vi "AFMss_control_trajTrack_deltaU_distEst.vi"() -> ()   [LabVIEW 2017]
uses:
  controls/controlParams_tracktraj.ctl
  <vilib>/rvi/Emulation/niFpgaGetClockAttributes.vi
  <vilib>/rvi/Emulation/niFpgaSctlEmulationGetInTimedLoop.vi
  <vilib>/rvi/Emulation/niFpgaEmulationReportErrorSimple.vi
  <vilib>/rvi/eio/common/nirviEmuTemplateMethod_errors.vi
  <vilib>/rvi/Emulation/niFpgaCriticalErrorInLSC.vi
  <vilib>/rvi/DataTransferAndStorage/Container/Common/niFpgaContainerExecOnDevCompGetState.vi
  <vilib>/rvi/Emulation/niFpgaEmulationIsFPGAContextNoSignature.vi
  <vilib>/rvi/DataTransferAndStorage/Container/Common/niFpgaContainerGetUniqueNameForEmu.vi
  <vilib>/rvi/Memory/Memory_Emulation/niFpgaMemoryEmulationCacheClearOnFirstRun.vi
  <vilib>/rvi/Memory/Memory_Emulation/nirvimemoryEmulationManagerCache_MakeExclusive.vi
  <vilib>/rvi/Memory/Memory_Emulation/niFpgaMemoryEmulationValidateCache.vi
  <vilib>/rvi/Memory/Memory_Emulation/nirvimemoryEmulationManagerCache_InsertValue.vi
  <vilib>/Utility/error.llb/Clear Errors.vi
  <vilib>/rvi/Memory/Memory_Emulation/nirvimemoryEmulationManagerCache_ReleaseExclusive.vi
  <vilib>/rvi/Memory/Memory_Emulation/nirvimemoryEmulationManagerCache_GetValue.vi
  <vilib>/rvi/Memory/Memory_Emulation/nirvimemoryEmulationManagerCache_SetValue.vi
  <vilib>/rvi/Emulation/niFpgaProcessEmulError.vi
  <vilib>/rvi/interface/RandomDataEmulation/niFpgaRandomDataHandleErrors.vi
  <vilib>/eio/EIONode/EIONode.xnode
  <vilib>/rvi/DataTransferAndStorage/Container/XNode/niFpgaContainer.xnode
  <vilib>/rvi/DataTransferAndStorage/Register/Emulation/niFpgaRegisterEmulationRefIn.vi
  <vilib>/rvi/interface/RandomDataEmulation/nirviRandomDataFpgaReadWriteTemplate.vi
  <vilib>/rvi/FXPMathLib/FxpSub/XNode/nifxpmath_Sub.xnode
  <vilib>/rvi/FXPMathLib/sim/FxpSim.dll
panel:
  in  "N_sat":i32
  in  "wsat_s":sgl[](array[numeric])=[0.0, 0.0, 0.0, 0.0, 0.0, 0.0, 0.0]
  in  "d_s":sgl[](array[numeric])=[0.0, 0.0, 0.0, 0.0, 0.0, 0.0, 0.0]
  in  "w_s":sgl[](array[numeric])=[0.0, 0.0, 0.0, 0.0, 0.0, 0.0, 0.0]
  in  "r_s":sgl[](array[numeric])=[0.0, 0.0, 0.0, 0.0, 0.0, 0.0, 0.0]
  in  "N_hyst":i32
  in  "Den":sgl[](array[numeric])=[0.982758, -1.98194, 1.0, 0.0, 0.0, 0.0, 0.0, 0.0, 0.0]
  in  "Num":sgl[](array[numeric])=[-0.00254, 0.000408, 0.00295, 0.0, 0.0, 0.0, 0.0, 0.0, 0.0]
  in  "TF Order":i32=2
  out "yk":sgl
  out "yuxk TO":bool
  out "YK TO":bool
  out "UK TO":bool
  in  "Cluster":T1={"umax"=3.0, "y_ref(k)"=0.0, "Ki"=0.0, "y(k) (from plant)"=0.0, "ND"=0, "NS"=0, "u_Kx_ref(k)"=0.0, "du_max"=3.0, "NS_obs"=0, "NS_control"=0, "Kp"=0.0} {"Kp" format="%#_13g"; "du_max" format="%#_13g"; "u_Kx_ref(k)" format="%#_13g"; "Ki" format="%#_13g"; "y_ref(k)" format="%#_13g"; "umax" format="%#_13g"}
  out "Unstable Traj":bool
  out "Loop Done":bool
  in  "Settle Ticks":i16=1000
  in  "False  = cont run":bool=TRUE
  in  "Abort":bool=TRUE
  in  "iters":i16=1
  in  "ymax":sgl=4.0 format="%#_13g"
  in  "TsTicks":i16
  out "Loop Ticks (benchmark)":i16
  out "NS_obs":i16=2
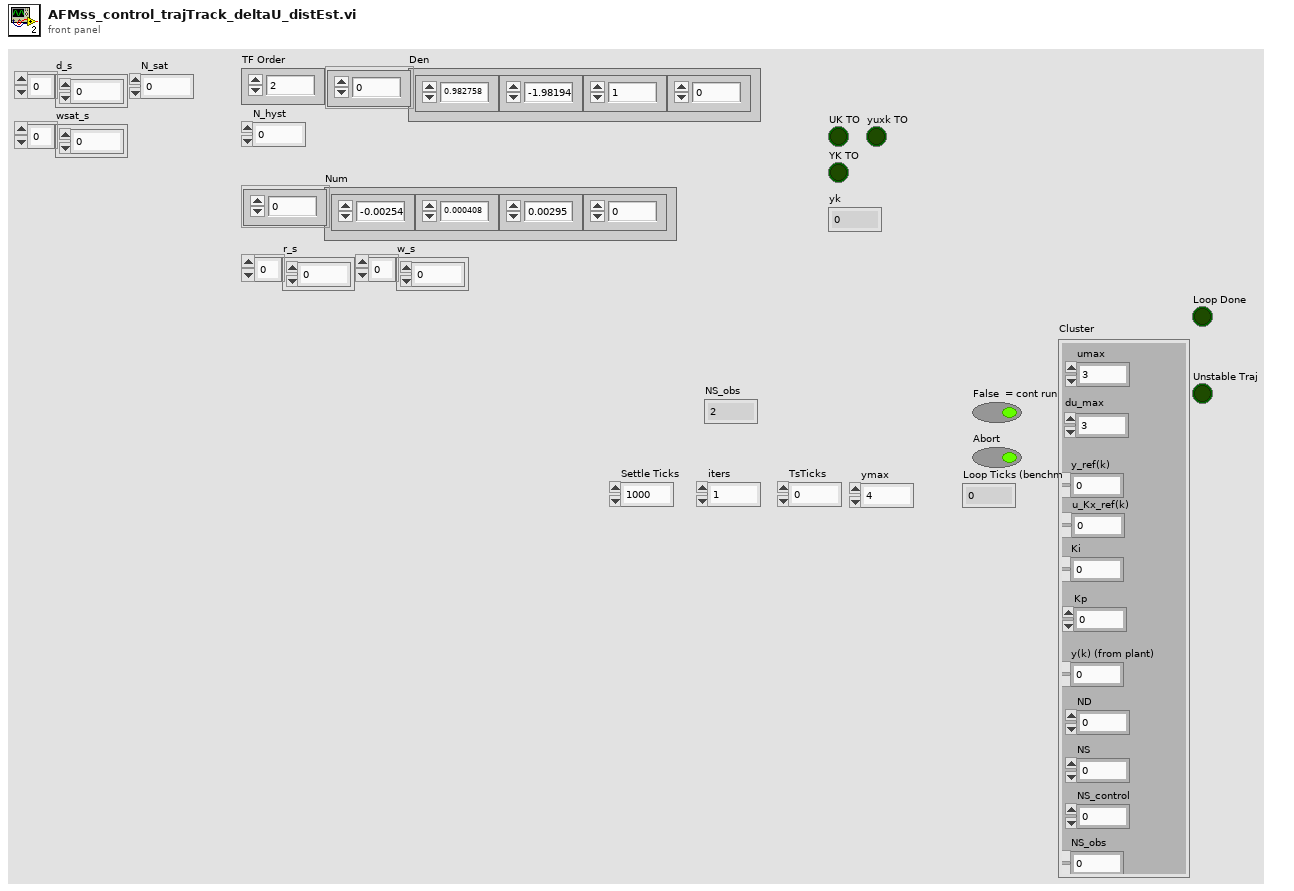
[diagram p1: front panel]
types:
  T1 = typedef "controlParams_tracktraj.ctl" = cluster{"umax":sgl, "y_ref(k)":sgl, "Ki":sgl, "y(k) (from plant)":sgl, "ND":i16, "NS":i16, "u_Kx_ref(k)":sgl, "du_max":sgl, "NS_obs":i16, "NS_control":i16, "Kp":sgl}
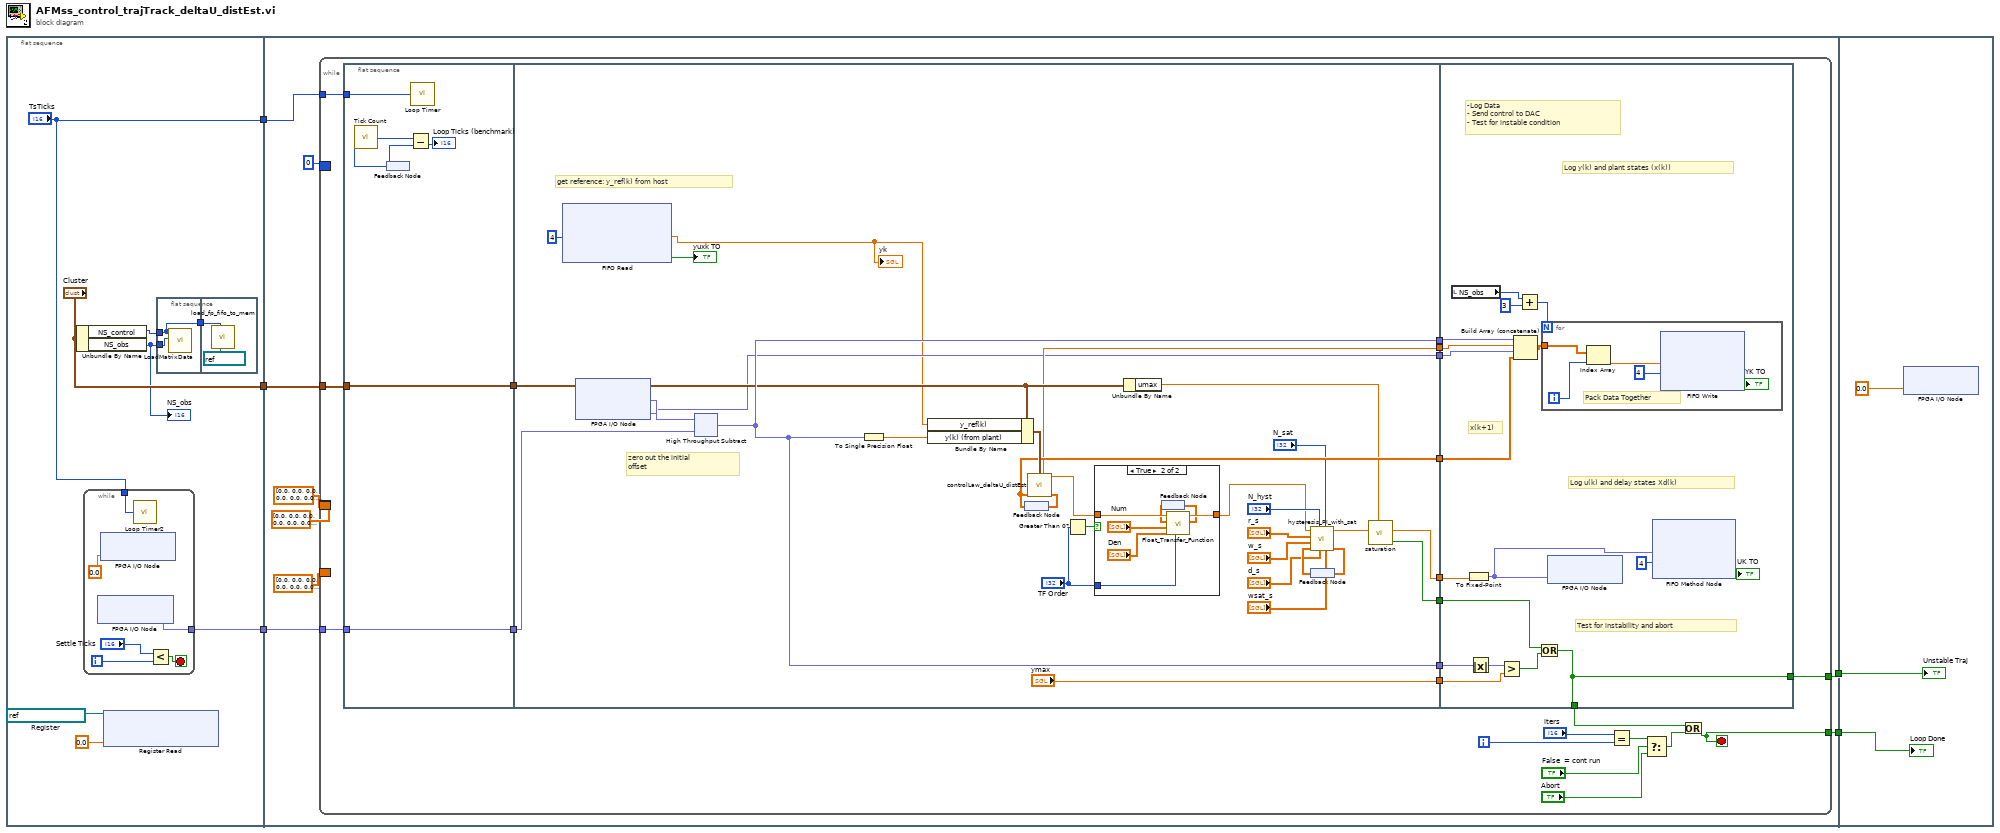
[diagram p0: block diagram]
diagram:
  n1 = flat-sequence {
    tunnel: ["TsTicks"] -> w5
    tunnel: [w13] -> w4
    tunnel: ["Cluster"] -> w2
    tunnel: w5 -> [w31]
    tunnel: w4 -> [w30]
    tunnel: [w29] -> w3
    tunnel: w2 -> [w28]
    tunnel: [w27] -> w1
    tunnel: w3 -> [w123]
    tunnel: w1 -> [w122]
    frame #0 {
      w11 = refnum<k21> "accumulator"  # Register
      # "Load Matrix Data"
      n2 = Unbundle By Name("Cluster") -> ("NS_control"=w8:i16, "NS_obs"=w6:i16)
      "NS_obs" <- w6
      n3 = while {
        tunnel: [w23] -> w13
        tunnel: "TsTicks" -> [w22]
        i -> [w18]
        stop <- w20 stop-if-true
        n4 = xnode "FPGA I/O Node"() -> ("Mod2/AI0"=w23:fxp<+/-,24,5>)  [unwired: 1 in, 1 out]
        n5 = xnode "FPGA I/O Node"("Mod1/AO0"=sgl 0.0) -> ()  [unwired: 1 in, 1 out]
        n6 = call "Loop Timer2"("Count(Ticks)"=w22) -> ()  [unwired: 1 out]
        n7 = Less?(x="Settle Ticks", y=w18) -> (x < y?=w20:bool)
      }
      n8 = xnode ("Register Read")("Data"=sgl 0.0, "Register In"=w11) -> ()  [unwired: 1 out]
      n9 = flat-sequence {
        tunnel: w8 -> [w15]
        tunnel: [w15] -> w7
        tunnel: w6 -> [w14]
        tunnel: w7 -> [w17]
        frame #0 {
          n10 = call "LoadMatrixData.vi"("NS_obs"=w14, "NS_control"=w15) -> ()  [unwired: 9 in, 1 out]
        }
        frame #1 {
          n11 = call "load_fp_fifo_to_mem.vi"("FP_memory"=refnum<k21> "Nx_x", "Len"=w17) -> ()  [unwired: 10 in]
        }
      }
    }
    frame #1 {
      n12 = while {
        border: i16 0 -> [_]
        tunnel: w31 -> [w46]
        tunnel: w30 -> [w44]
        tunnel: [w42] -> w29
        tunnel: w28 -> [w40]
        tunnel: [w39] -> w27
        border: sgl[] [0.0, 0.0, 0.0, 0.0, 0.0, 0.0, 0.0, 0.0, 0.0] ("State Out") -> [_]
        border: sgl[] [0.0, 0.0, 0.0, 0.0, 0.0, 0.0, 0.0] ("y_vec_out") -> [_]
        border: sgl[] [0.0, 0.0, 0.0, 0.0, 0.0, 0.0, 0.0, 0.0, 0.0, 0.0, 0.0, 0.0, 0.0, 0.0, 0.0, 0.0, 0.0, 0.0, 0.0, 0.0, 0.0, 0.0, 0.0, 0.0, 0.0] ("x^(k+1) = Ax + Bu + Lye") -> [_]
        i -> [w51]
        stop <- w42 stop-if-true
        n13 = flat-sequence {
          tunnel: w46 -> [w57]
          tunnel: w44 -> [w56]
          tunnel: [w56] -> w43
          tunnel: [w55] -> w41
          tunnel: w40 -> [w55]
          tunnel: [w63] -> w54
          tunnel: [w88] -> w45
          tunnel: w43 -> [w90]
          tunnel: w41 -> [w87]
          tunnel: [w75] -> w38
          tunnel: [w88] -> w37
          tunnel: ["ymax"] -> w36
          tunnel: [w71] -> w35
          tunnel: [w70] -> w34
          tunnel: [w62] -> w33
          tunnel: w54 -> [w110]
          tunnel: [w107] -> w53
          tunnel: w45 -> [w106]
          tunnel: [w107] -> w39
          tunnel: w38 -> [w105]
          tunnel: w37 -> [w114]
          tunnel: w36 -> [w109]
          tunnel: w35 -> [w101]
          tunnel: w34 -> [w100]
          tunnel: w33 -> [w99]
          frame #0 {
            n14 = call "Tick Count"() -> ("Tick Count(Ticks)"=w58:u32)
            n15 = feedback #1() -> (w59:u32)
            n16 = feedback-in #1(w58) -> ()
            n17 = Subtract(x=w58, y=w59) -> (x-y=→"Loop Ticks (benchmark)":u32)
            n18 = call "Loop Timer"("Count(Ticks)"=w57) -> ()  [unwired: 1 out]
          }
          frame #1 {
            # "get reference: y_ref(k) from host"
            # "zero out the initial \noffset"
            n19 = xnode ("FIFO Read")("Timeout"=i16 4) -> ("Element"=w67:sgl, "Timed Out?"=→"yuxk TO":bool)  [unwired: 1 in, 1 out]
            "yk" <- w67
            n20 = xnode "FPGA I/O Node"() -> ("Mod2/AI0"=w85:fxp<+/-,24,5>, "Mod2/AI2"=w70:fxp<+/-,24,5>)  [unwired: 2 in, 2 out]
            n21 = xnode "High Throughput Subtract"("x"=w85, "y"=w90) -> ("x-y"=w88:fxp<+/-,40,6>)
            n22 = To Single Precision Float(number=w88) -> (single precision float=w89:sgl)
            n23 = Bundle By Name(cluster=w87, "y_ref(k)"=w67, "y(k) (from plant)"=w89) -> (w77:T1)
            n24 = feedback #2() -> (w75:sgl[])
            n25 = call "controlLaw_deltaU_distEst.vi"("Control Params"=w77, "x^(k)"=w75) -> ("x^(k+1) = Ax + Bu + Lye"=w76:sgl[], "u(k) (unsaturated)"=w66:sgl, "delta u(k)"=w71:sgl)  [unwired: 7 in]
            n26 = feedback-in #2(w76) -> ()
            n27 = Greater Than 0?(x="TF Order") -> (x > 0?=w84:bool)
            n28 = case shown="True" w84 {
              tunnel: w66 -> [w91 w98]
              tunnel: "TF Order" -> [_ w97]
              tunnel: [w91 w96] -> w65
              frame False {
              }
              frame True {
                n29 = feedback #3() -> (w94:sgl[])
                n30 = call "Float_Transfer_Function.vi"("TF Order"=w97, "Den"="Den", "Num"="Num", "State In"=w94, "Input"=w98) -> ("State Out"=w95:sgl[], "Output"=w96:sgl)  [unwired: 4 in]
                n31 = feedback-in #3(w95) -> ()
              }
            }
            n32 = Unbundle By Name(w87) -> ("umax"=w61:sgl)
            n33 = feedback #4() -> (w81:sgl[])
            n34 = call "hysteresis_PI_with_sat.vi"("wsat_s"="wsat_s", "N_sat"="N_sat", "d_s"="d_s", "N_hyst"="N_hyst", "y_vec_in"=w81, "w_s"="w_s", "r_s"="r_s", "uk"=w65) -> ("y_vec_out"=w82:sgl[], "H_of_ik"=w64:sgl)  [unwired: 2 in]
            n35 = feedback-in #4(w82) -> ()
            n36 = call "saturation.vi"("uMax"=w61, "signal in"=w64) -> ("has_saturated"=w62:bool, "signal out"=w63:sgl)  [unwired: 8 in]
          }
          frame #2 {
            # "x(k+1)"
            # "Log u(k) and delay states Xd(k)"
            # "Log y(k) and plant states (x(k))"
            # "-Log Data\n- Send control to DAC\n- Test for instable condition"
            # "Test for instability and abort"
            n37 = local read "NS_obs"() -> (w103:i16)
            n38 = To Fixed-Point(number=w110) -> (fixed-point=w113:fxp<+/-,32,6>)  [unwired: 1 in]
            n39 = Absolute Value(x=w114) -> (abs(x)=w116:fxp<+,40,6>)
            n40 = Greater?(x=w116, y=w109) -> (0:w108:bool)
            n41 = Build Array (concatenate)(w106, w101, w100, w105) -> (w115:sgl[])
            n42 = Add(x=w103, y=i16 3) -> (x+y=w104:i16)
            n43 = Or(x=w99, y=w108) -> (x .or. y?=w107:bool)
            n44 = for {
              N: w104 -> [_]
              tunnel: w115 -> [w119]
              i -> [w120]
              # "Pack Data Together"
              n45 = Index Array(array=w119, index=w120) -> (element=w118:sgl)
              n46 = xnode ("FIFO Write")("Element"=w118, "Timeout"=i16 4) -> ("Timed Out?"=→"YK TO":bool)  [unwired: 1 in, 1 out]
            }
            n47 = xnode "FPGA I/O Node"("Mod1/AO0"=w113) -> ()  [unwired: 1 in, 1 out]
            n48 = xnode ("FIFO Method Node")("Element"=w113, "Timeout"=i16 4) -> ("Timed Out?"=→"UK TO":bool)  [unwired: 1 in, 1 out]
          }
        }
        n49 = Equal?(x="iters", y=w51) -> (x = y?=w49:bool)
        n50 = Select(t=w49, s="False  = cont run", f="Abort") -> (s? t:f=w50:bool)
        n51 = Or(x=w53, y=w50) -> (x .or. y?=w42:bool)
      }
    }
    frame #2 {
      n52 = xnode "FPGA I/O Node"("Mod1/AO0"=sgl 0.0) -> ()  [unwired: 1 in, 1 out]
      "Loop Done" <- w123
      "Unstable Traj" <- w122
    }
  }
